vi "tmp_toml_fg.vi"(7 "cmd":string, 8 "error in (no error)":errorcluster, 10 "data in":variant, 11 "path in":path) -> (0 "error out":errorcluster, 1 "exists":bool, 2 "data out":variant, 3 "files":path[](array[path]))   [LabVIEW 2017]
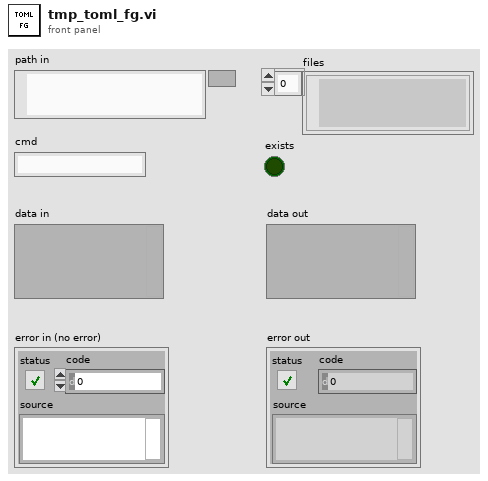
[diagram p1: front panel]
types:
  T1 = enum16{"open", "replace", "create", "open or create", "replace or create", "replace or create with confirmation"}
  T2 = cluster{"section":string, "key":string, "value":variant}
  T3 = cluster{"s":string, "#":string, "..":string, "kv#p":string[][]}[]
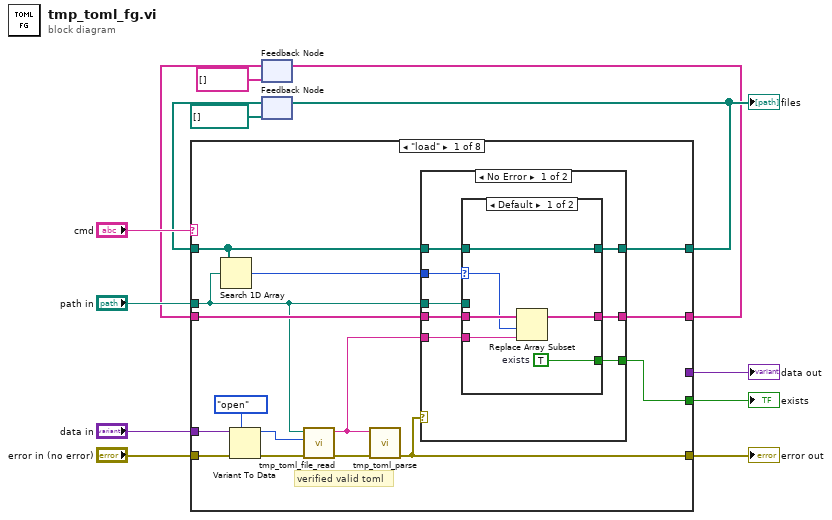
[diagram p0: block diagram]
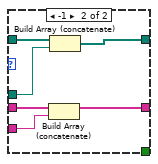
[diagram p2: hidden frame]
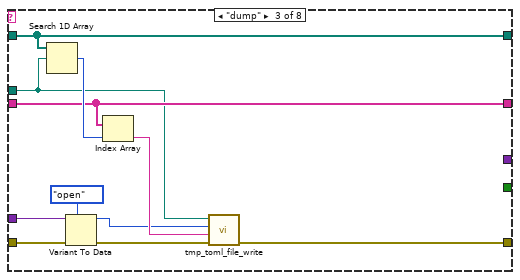
[diagram p5: hidden frame]
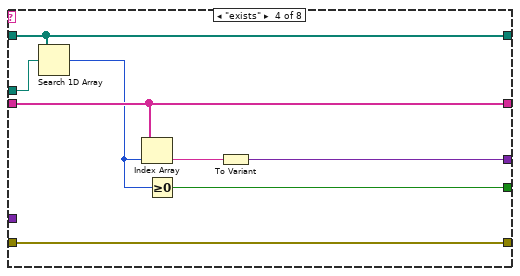
[diagram p6: hidden frame]
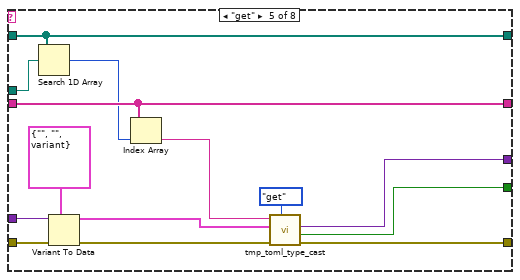
[diagram p7: hidden frame]
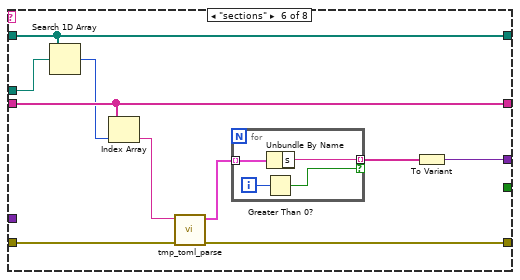
[diagram p8: hidden frame]
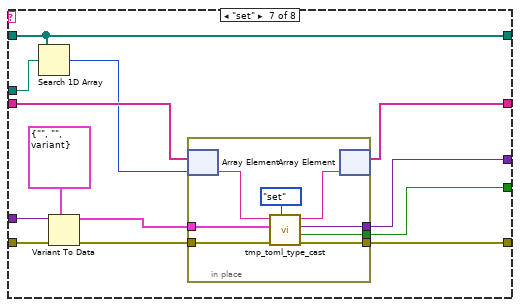
[diagram p9: hidden frame]
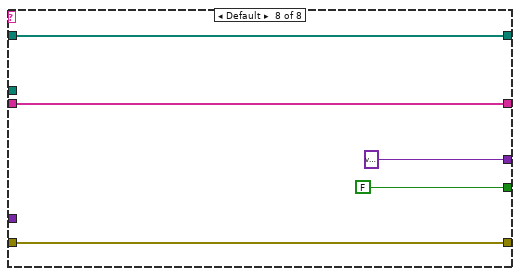
[diagram p10: hidden frame]
diagram:
  n1 = feedback #1(string[] []) -> (w4:string[])
  n2 = feedback #2(path[] []) -> (w8:path[])
  n3 = case shown="\"load\"" "cmd" {
    tunnel: [w14 w53 w60 w70 w78 w90 w107 w126] -> w12
    tunnel: "error in (no error)" -> [w25 w53 w61 w70 w84 w91 w111 w126]
    tunnel: "path in" -> [w19 _ w59 w71 w85 w95 w112 _]
    tunnel: w8 -> [w28 w52 w64 w72 w86 w96 w113 w124]
    tunnel: [w21 w52 w64 w72 w86 w96 w113 w124] -> w7
    tunnel: [w26 w51 w62 w68 w83 w94 w101 w125] -> w5
    tunnel: w4 -> [w27 w51 w62 w68 w83 w94 w103 w125]
    tunnel: "data in" -> [w24 _ w56 _ w81 _ w110 _]
    tunnel: [_ _ _ w65 w74 w92 w105 variant] -> w2
    tunnel: [w18 _ _ w69 w73 _ w104 FALSE] -> w1
    frame "load" {
      # "verified valid toml"
      n4 = Search 1D Array(1D array=w28, element=w19) -> (index of element=w20:i32)  [unwired: 1 in]
      n5 = Variant To Data(error in=w25, type=T1."open" ("operation"), Variant=w24) -> (data=w22:T1, error out=w23:errorcluster)
      n6 = call "tmp_toml_file_read.vi"("error in (no error)"=w23, "operation (open or create)"=w22, "path"=w19) -> ("error out"=w16:errorcluster, "text"=w15:string)  [unwired: 7 in]
      n7 = call "tmp_toml_parse.vi"("error in (no error)"=w16, "text in"=w15) -> ("error out"=w14:errorcluster)  [unwired: 8 in, 1 out]
      n8 = case shown="No Error" w14 {
        tunnel: w28 -> [w36 w50]
        tunnel: w27 -> [w35 w49]
        tunnel: [w34 w49] -> w26
        tunnel: [w33 w50] -> w21
        tunnel: w20 -> [w32 _]
        tunnel: w19 -> [w31 _]
        tunnel: [w30 _] -> w18
        tunnel: w15 -> [w29 _]
        frame No Error {
          n9 = case shown="Default" w32 {
            selector: w32 -> [w37 _]
            tunnel: w36 -> [w42 w48]
            tunnel: w35 -> [w41 w47]
            tunnel: [w40 w46] -> w34
            tunnel: w29 -> [w39 w45]
            tunnel: [w42 w44] -> w33
            tunnel: w31 -> [_ w43]
            tunnel: [w38 _] -> w30
            frame Default {
              w38 = TRUE  # exists
              n10 = Replace Array Subset(array=w41, new element=w39, index=w37) -> (w40:string[])
            }
            frame -1 {
              n11 = Build Array (concatenate)(w47, w45) -> (w46:string[])
              n12 = Build Array (concatenate)(w48, w43) -> (w44:path[])
            }
          }
        }
        frame Error {
        }
      }
    }
    frame "null" {
    }
    frame "dump" {
      n13 = Search 1D Array(1D array=w64, element=w59) -> (index of element=w63:i32)  [unwired: 1 in]
      n14 = Variant To Data(error in=w61, type=T1."open" ("operation (replace or create)"), Variant=w56) -> (data=w54:T1, error out=w57:errorcluster)
      n15 = Index Array(array=w62, index=w63) -> (element=w58:string)
      n16 = call "tmp_toml_file_write.vi"("error in (no error)"=w57, "text"=w58, "operation (replace or create)"=w54, "path"=w59) -> ("error out"=w60:errorcluster)  [unwired: 7 in]
    }
    frame "exists" {
      n17 = Search 1D Array(1D array=w72, element=w71) -> (index of element=w67:i32)  [unwired: 1 in]
      n18 = Index Array(array=w68, index=w67) -> (element=w66:string)
      n19 = Greater Or Equal To 0?(x=w67) -> (x >= 0?=w69:bool)
      n20 = To Variant(anything=w66) -> (Variant=w65:variant)
    }
    frame "get" {
      n21 = Search 1D Array(1D array=w86, element=w85) -> (index of element=w82:i32)  [unwired: 1 in]
      n22 = Variant To Data(error in=w84, type=T2 {"section"="", "key"="", "value"=variant} ("item"), Variant=w81) -> (data=w76:T2, error out=w79:errorcluster)
      n23 = Index Array(array=w83, index=w82) -> (element=w77:string)
      n24 = call "tmp_toml_type_cast.vi"("action"=enum8{"get", "set"}."get", "error in (no error)"=w79, "item"=w76, "text in"=w77) -> ("error out"=w78:errorcluster, "exists?"=w73:bool, "value"=w74:variant)  [unwired: 4 in, 1 out]
    }
    frame "sections" {
      n25 = Search 1D Array(1D array=w96, element=w95) -> (index of element=w93:i32)  [unwired: 1 in]
      n26 = Index Array(array=w94, index=w93) -> (element=w89:string)
      n27 = call "tmp_toml_parse.vi"("error in (no error)"=w91, "text in"=w89) -> ("error out"=w90:errorcluster, "sections"=w88:T3)  [unwired: 8 in]
      n28 = for {
        tunnel: w88 -> [w100] mode=indexing
        tunnel: [w99] -> w87 mode=indexing if=w97
        i -> [w98]
        n29 = Greater Than 0?(x=w98) -> (x > 0?=w97:bool)
        n30 = Unbundle By Name(w100) -> ("s"=w99:string)
      }
      n31 = To Variant(anything=w87) -> (Variant=w92:variant)
    }
    frame "set" {
      n32 = Search 1D Array(1D array=w113, element=w112) -> (index of element=w102:i32)  [unwired: 1 in]
      n33 = Variant To Data(error in=w111, type=T2 {"section"="", "key"="", "value"=variant} ("item"), Variant=w110) -> (data=w106:T2, error out=w108:errorcluster)
      n34 = in-place {
        in-place-border: w108 -> [w121]
        in-place-border: [w120] -> w107
        in-place-border: w106 -> [w119]
        in-place-border: [w117] -> w105
        in-place-border: [w116] -> w104
        n35 = in-place-array #3(w103, w102) -> (w115:string)
        n36 = call "tmp_toml_type_cast.vi"("action"=enum8{"get", "set"}."set", "error in (no error)"=w121, "item"=w119, "text in"=w115) -> ("error out"=w120:errorcluster, "exists?"=w116:bool, "value"=w117:variant, "text out"=w114:string)  [unwired: 4 in]
        n37 = in-place-array #3(w114) -> (w101:string[])  [unwired: 1 out]
      }
    }
    frame Default {
    }
  }
  "error out" <- w12
  "data out" <- w2
  "files" <- w7
  "exists" <- w1
  n38 = feedback-in #1(w5) -> ()
  n39 = feedback-in #2(w7) -> ()
